vi "Modified JSON Variant Tools.vi"() -> ()   [LabVIEW 2011]
doc: "Demonstrates the use of the Variant JSON VIs for converting to and from a complex cluster."
uses:
  JSON Scalar/Infinity&NaN.ctl
  JSON Value/Set from JSON string.vi
  Variant JSON/Variant to JSON.vi
  JSON Value/Get as JSON string (pretty).vi
  Variant JSON/Get as Variant.vi
  JSON Value/JSON Value.lvclass
  Get Polymorphic/JSON GetSet.lvlib
  Variant JSON/Variant JSON.lvlib
  JSON Scalar/JSON Scalar.lvclass
panel:
  in  "Treatment of Infinity/NaN":T1
  out "Time":dbl format="%#_6p"
  out "error out":errorcluster
  out "Variant after setting":variant
  out "Cluster after setting":T2={"T1"=0.0, "Nest"={"NestNest"={"A"="", "Complex"=0.0+0.0i, "C"=0.0}, "Enum"=enum."AAA"}, "Test Array"=[], "Boolean 1"=FALSE, "T2"="", "Boolean 2"=FALSE, "Time Stamp"=timestamp(0 s since 1904-01-01), "Infinity"=0.0, "NAN"=0.0, "TTT"=0.0, "waveform"={"t0"=timestamp(0 s since 1904-01-01), "dt"=1.0, "Y"=[]}, "Test Array 2D"=[], "String Array"=[["", "", ""]], "Path"=path "", "App Refnum"=refnum}
  in  "Cluster to set":T2={"T1"=0.0, "Nest"={"NestNest"={"A"="", "Complex"=0.0+0.0i, "C"=0.0}, "Enum"=enum."AAA"}, "Test Array"=[], "Boolean 1"=FALSE, "T2"="", "Boolean 2"=FALSE, "Time Stamp"=timestamp(0 s since 1904-01-01), "Infinity"=0.0, "NAN"=0.0, "TTT"=0.0, "waveform"={"t0"=timestamp(0 s since 1904-01-01), "dt"=1.0, "Y"=[]}, "Test Array 2D"=[], "String Array"=[["", "", ""]], "Path"=path "", "App Refnum"=refnum}
  in  "Creation cluster":T3={"T2"="Test \"quote\",\nand newline.", "Nest"={"Enum"=enum."CCC (with a space)", "NestNest"={"A"=34.0, "Complex"=2.0+3.1i, "C"="1.23 string"}}, "Test Array"=[456.789, 2.0, 3.0], "Boolean 1"=TRUE, "T1"=456.789, "Boolean 2"="true (a string)", "Time Stamp"=timestamp(3434102896.3125 s since 1904-01-01), "Extra item"="test2", "Infinity"=inf, "NAN"=nan, "TTT"="any non number", "waveform"={"t0"=timestamp(3436250625 s since 1904-01-01), "dt"=1.0, "Y"=[23.0, 34.0]}, "Test Array 2D"=[[1.0, 2.0], [3.0, 4.0], [5.0, 6.0], [7.0, 8.0]], "String Array"=[["one", "number 2", "three"], ["1one", "two", "3"]], "Path"=path "c:/temp123.txt", "App Refnum"=refnum}
  out "JSON String created":string
  # "see diagram"
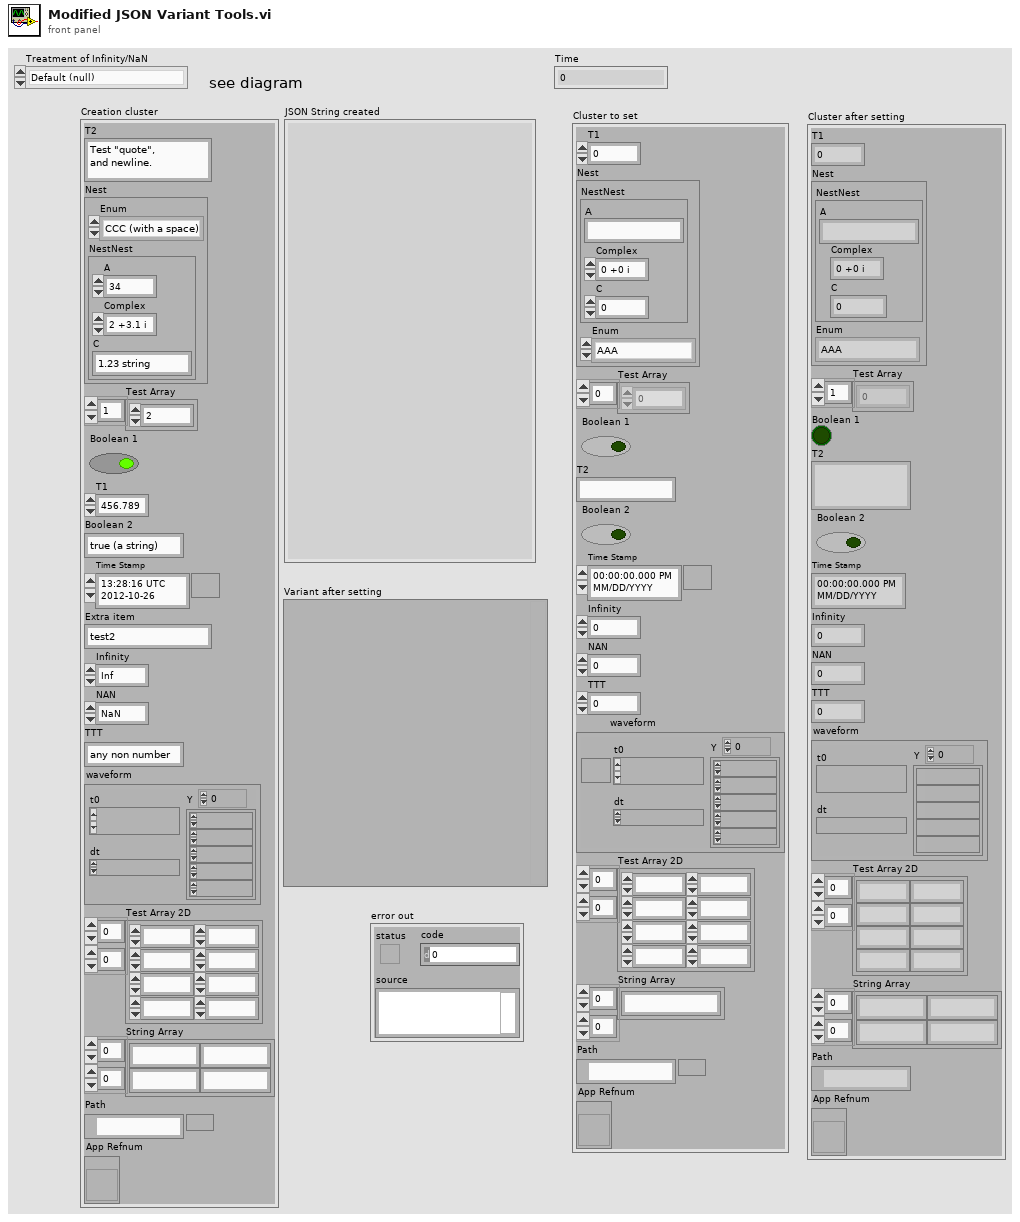
[diagram p1: front panel]
types:
  T1 = typedef "JSON Scalar.lvclass/Infinity&NaN.ctl" = enum16{"Default (null)", "Extended", "LabVIEW extensions"}
  T2 = cluster{"T1":dbl, "Nest":cluster{"NestNest":cluster{"A":string, "Complex":cdb, "C":dbl}, "Enum":enum16{"AAA", "BBB", "CCC (with a space)"}}, "Test Array":dbl[], "Boolean 1":bool, "T2":string, "Boolean 2":bool, "Time Stamp":timestamp, "Infinity":dbl, "NAN":dbl, "TTT":dbl, "waveform":waveform(dbl), "Test Array 2D":dbl[][], "String Array":string[][], "Path":path, "App Refnum":refnum<vi>}
  T3 = cluster{"T2":string, "Nest":cluster{"Enum":enum16{"AAA", "BBB", "CCC (with a space)"}, "NestNest":cluster{"A":dbl, "Complex":cdb, "C":string}}, "Test Array":dbl[], "Boolean 1":bool, "T1":dbl, "Boolean 2":string, "Time Stamp":timestamp, "Extra item":string, "Infinity":dbl, "NAN":dbl, "TTT":string, "waveform":waveform(dbl), "Test Array 2D":dbl[][], "String Array":string[][], "Path":path, "App Refnum":refnum<vi>}
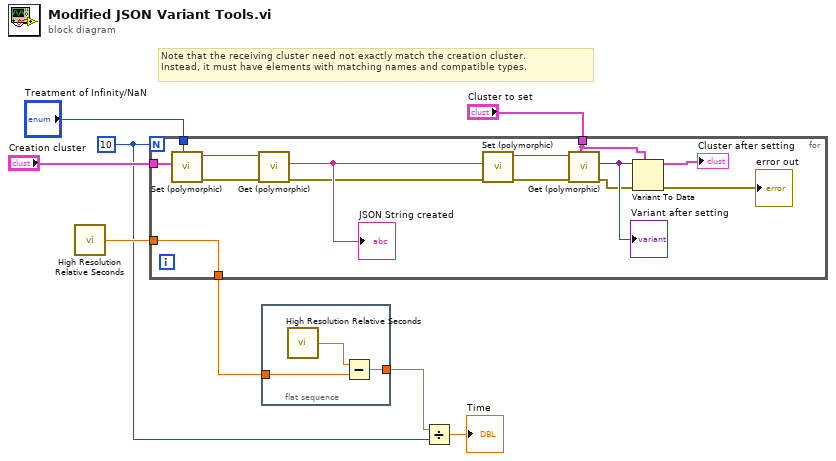
[diagram p0: block diagram]
diagram:
  w3 = 10
  # "Note that the receiving cluster need not exactly match the creation cluster.\nInstead, it must have elements with matching names and compatible types."
  n1 = call <vilib>:"High Resolution Relative Seconds.vi"() -> ("relative seconds"=w6:dbl)
  n2 = for {
    N: w3 -> [_]
    tunnel: "Creation cluster" -> [w14]
    tunnel: "Cluster to set" -> [w12]
    tunnel: w6 -> [w10]
    tunnel: [w10] -> w5
    tunnel: "Treatment of Infinity/NaN" -> [w9]
    n3 = call-poly "Set (polymorphic).vi"("Treatment of Infinity/NaN"=w9, "Variant"=w14) -> ("error out"=w17:errorcluster, "JSON Value out"=w22:refnum<class "JSON Value.lvclass">)  [unwired: 8 in]
    n4 = call-poly "Get (polymorphic).vi"("error in (no error)"=w17, "JSON Value in"=w22) -> ("error out"=w16:errorcluster, "String"=w18:string)  [unwired: 8 in]
    "JSON String created" <- w18
    n5 = call-poly "Set (polymorphic).vi"("error in (no error)"=w16, "JSON stream"=w18) -> ("error out"=w13:errorcluster, "JSON Value out"=w15:refnum<class "JSON Value.lvclass">)  [unwired: 7 in, 1 out]
    n6 = call-poly "Get (polymorphic).vi"("Variant (Data Type)"=w12, "error in (no error)"=w13, "JSON in"=w15) -> ("error out"=w19:errorcluster, "Variant out"=w21:variant)  [unwired: 6 in, 1 out]
    "Variant after setting" <- w21
    n7 = Variant To Data(error in=w19, type=w12, Variant=w21) -> (data=→"Cluster after setting":T2, error out=→"error out":errorcluster)
  }
  n8 = flat-sequence {
    tunnel: w5 -> [w24]
    tunnel: [w23] -> w4
    frame #0 {
      n9 = call <vilib>:"High Resolution Relative Seconds.vi"() -> ("relative seconds"=w25:dbl)
      n10 = Subtract(x=w25, y=w24) -> (x-y=w23:dbl)
    }
  }
  n11 = Divide(x=w4, y=w3) -> (x/y=→"Time":dbl)
